vi "Read Lower Limit.vi"(8 "error in (no error)":errorcluster, 11 "Test Double Float in":refnum<class "Test Double Float.lvclass">) -> (0 "error out":errorcluster, 2 "Lower Limit":dbl, 3 "Test Double Float out":refnum<class "Test Double Float.lvclass">)   [LabVIEW 2021, in "BT.lvlib" / "Test Double Float.lvclass"]
uses:
  Test Double Float.lvclass
  Test Double Float.lvclass/Test Double Float.ctl
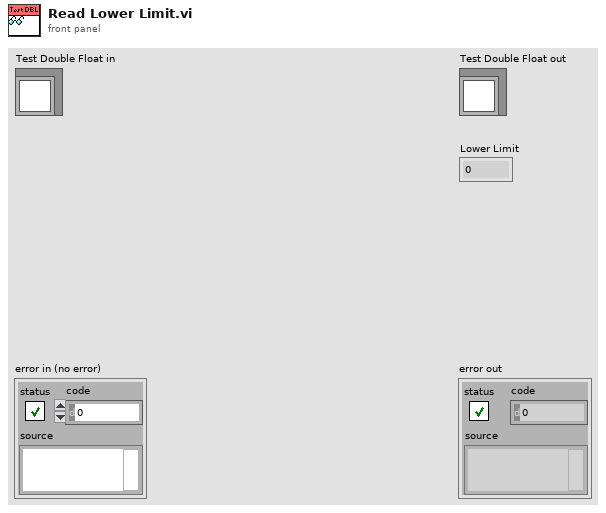
[diagram p1: front panel]
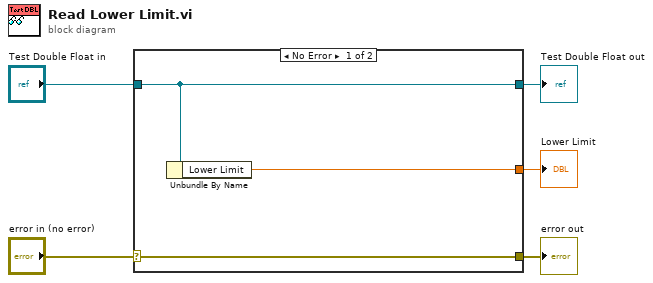
[diagram p0: block diagram]
diagram:
  n1 = case shown="No Error" "error in (no error)" {
    selector: "error in (no error)" -> [w8 w9]
    tunnel: [w8 w9] -> w4
    tunnel: [w7 w10] -> w2
    tunnel: "Test Double Float in" -> [w7 w10]
    tunnel: [w6 _] -> w1
    frame No Error {
      n2 = Unbundle By Name(w7) -> ("Lower Limit"=w6:dbl)
    }
    frame Error {
    }
  }
  "error out" <- w4
  "Test Double Float out" <- w2
  "Lower Limit" <- w1
